vi "lab project final (3).vi"() -> ()   [LabVIEW 2010]
doc: "Use this template to simulate the generation and display of data.\nNote: LabVIEW enables automatic error handling by default for VIs you create from this template."
uses:
  <vilib>/Analysis/4window.llb/windowTd.ctl
  <vilib>/express/express arith-compare/Formula/XNode/ExpressFormulaBlockNode.xnode
  <vilib>/measure/maspectr.llb/FFT Spectrum (Mag-Phase) for 1 Chan.vi
  <vilib>/measure/NI_MAPro.lvlib
  <vilib>/measure/NI_MABase.lvlib
  <vilib>/Analysis/NI_AALPro.lvlib
panel:
  out "Previous":dbl
  out "Result":dbl
  in  "Previous Peak":bool
  in  "Next Peak":bool
  in  "Numeric":dbl
  in  "Span":dbl
  in  "Frequency":dbl
  out "Spectrum Analysis":cluster{"f0":dbl, "df":dbl, "magnitude":dbl[]}(graph)
  in  "Manual Mode":bool
  in  "Number of Cycles":i32(knob) scale=1.0..7.0
  in  "Offset":dbl(knob) scale=0.0..10.0
  in  "signal type":T1(ring)
  in  "Phase":dbl(knob) scale=0.0..10.0
  in  "Frequency":dbl(knob) scale=0.0..10000.0
  in  "Amplitude":dbl(knob) scale=0.0..10.0
  out "Waveform Graph 2":waveform(dbl)(graph)
  in  "window":T2=1 items=["Rectangle"=0, "Hanning"=1, "Hamming"=2, "Blackman-Harris"=3, "Exact Blackman"=4, "Blackman"=5, "Flat Top"=6, "4 Term B-Harris "=7, "7 Term B-Harris"=8, "Low Sidelobe"=9, "Blackman Nuttall"=11, "Triangle"=30, "Bartlett-Hanning"=31, "Bohman"=32, "Parzen"=33, "Welch"=34, "Kaiser"=60, "Dolph-Chebyshev"=61, "Gaussian"=62]
  in  "averaging parameters":T3={"averaging mode"=enum."No averaging", "weighting mode"=enum."Exponential", "number of averages"=10} {"number of averages" min=1}
  out "averaging done":bool
  out "averages completed":dbl
  in  "restart averaging (F)":bool
  in  "view":T4
  in  "stop":bool
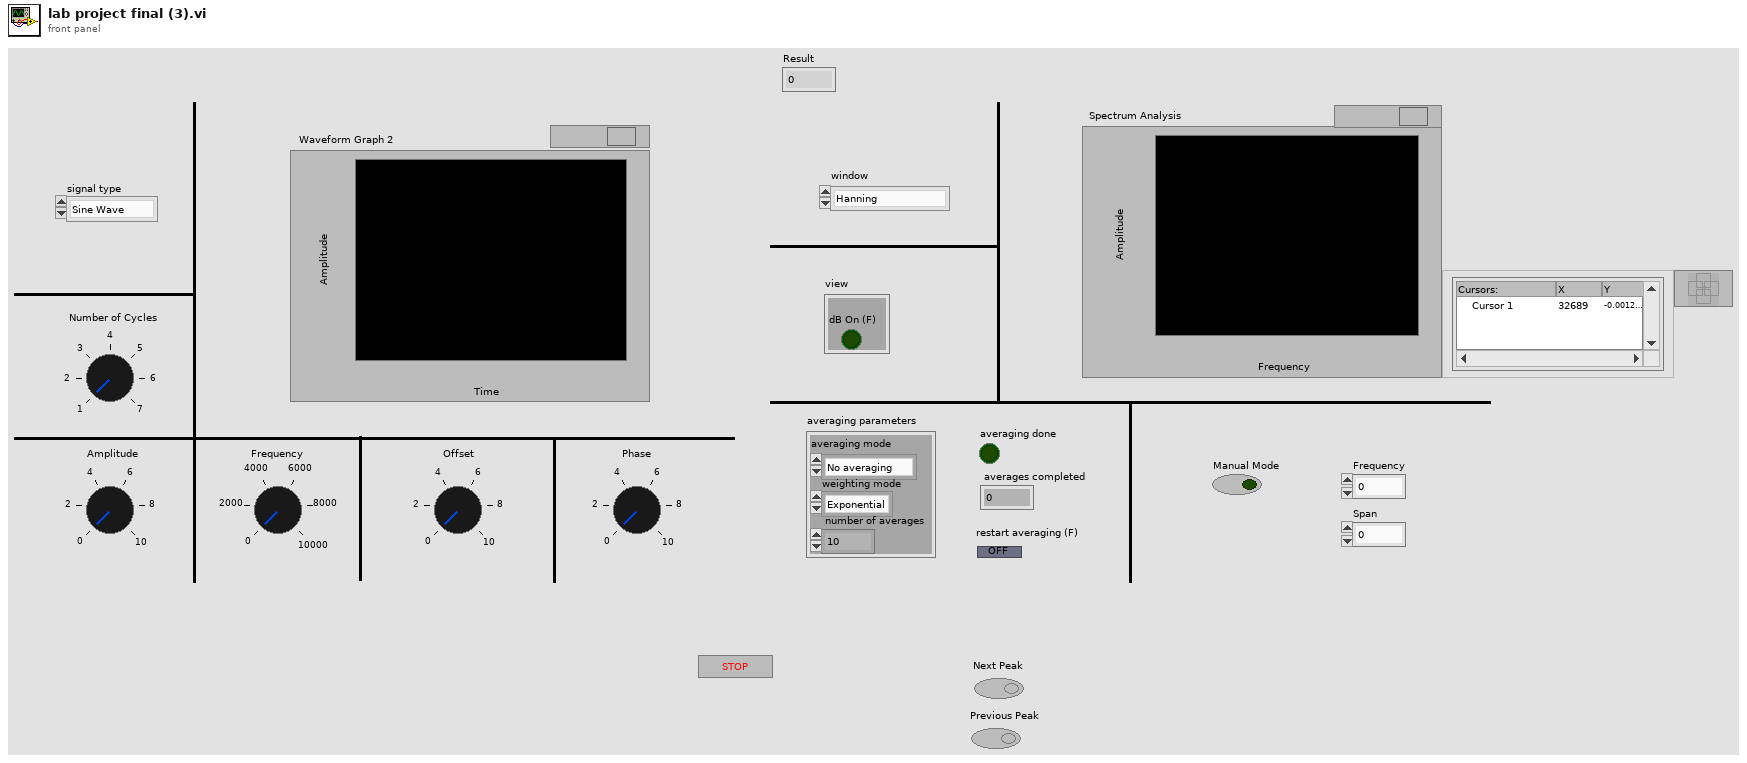
[diagram p1: front panel]
types:
  T1 = enum16{"Sine Wave", "Triangle Wave", "Square Wave", "Sawtooth Wave"}
  T2 = typedef "NI_AALPro.lvlib/windowTd.ctl" = u32
  T3 = cluster{"averaging mode":enum16{"No averaging", "Vector averaging", "RMS averaging", "Peak hold"}, "weighting mode":enum16{"Linear", "Exponential"}, "number of averages":u32}
  T4 = cluster{"dB On (F)":bool, "unwrap phase (F)":bool, "convert to degree (F)":bool}
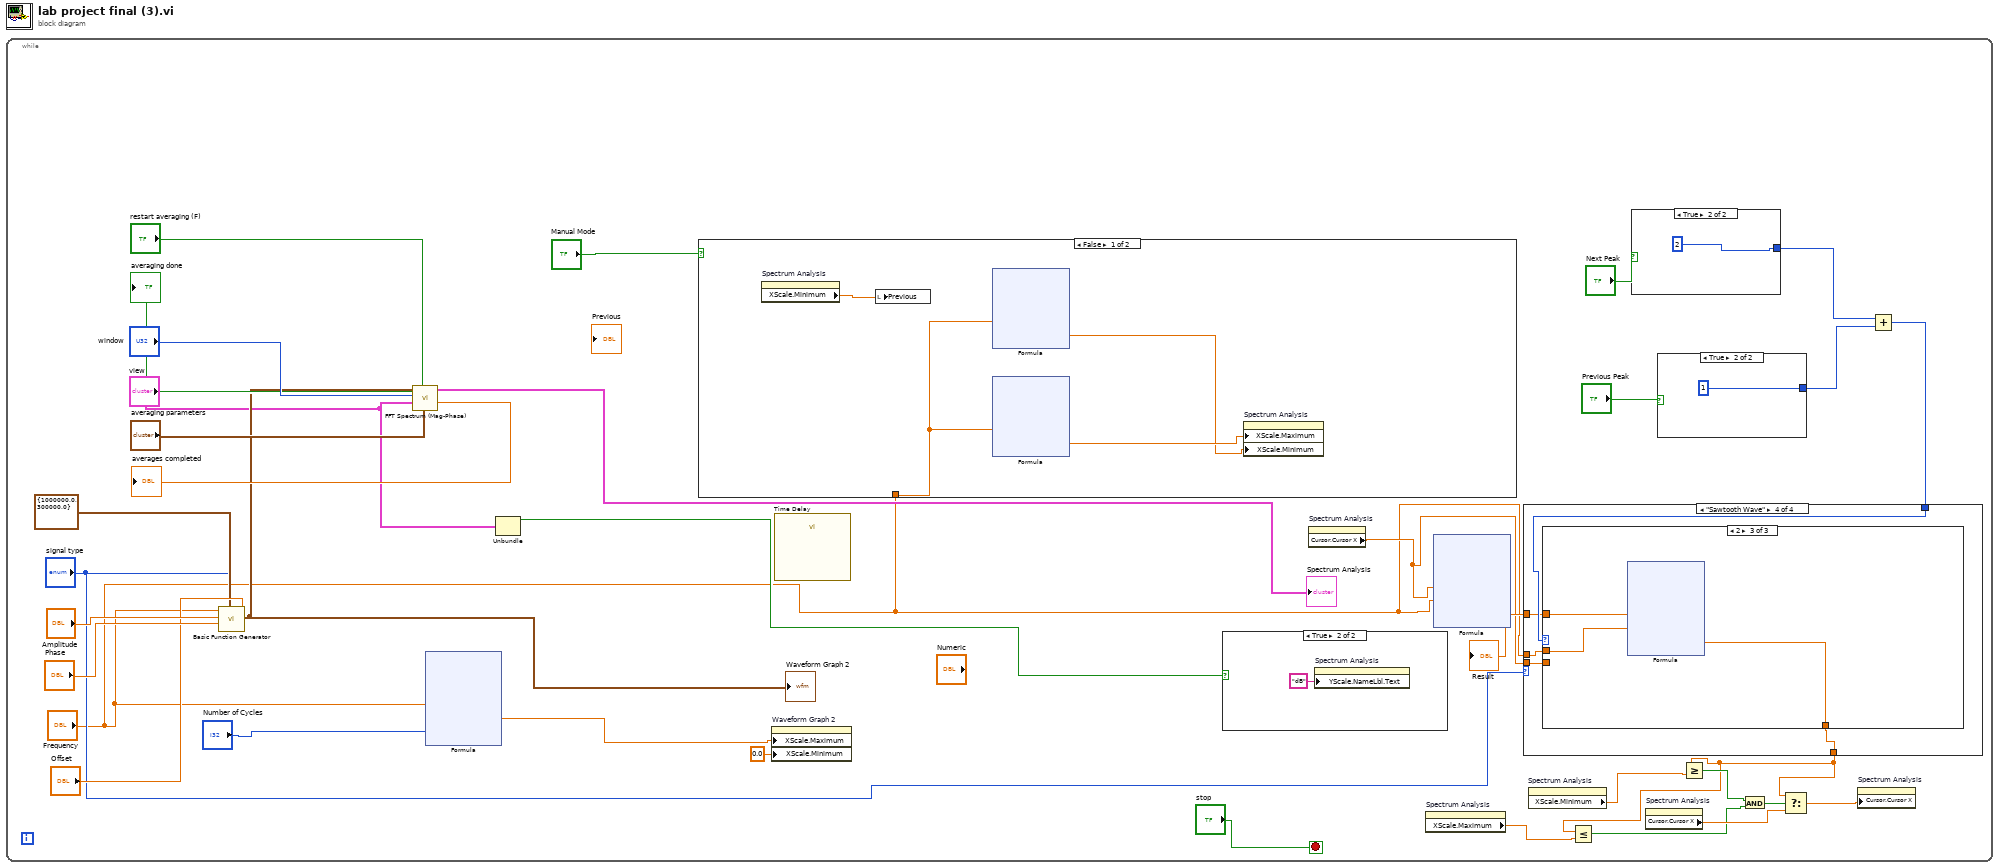
[diagram p0: block diagram]
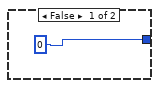
[diagram p2: hidden frame]
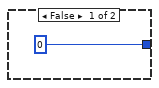
[diagram p3: hidden frame]
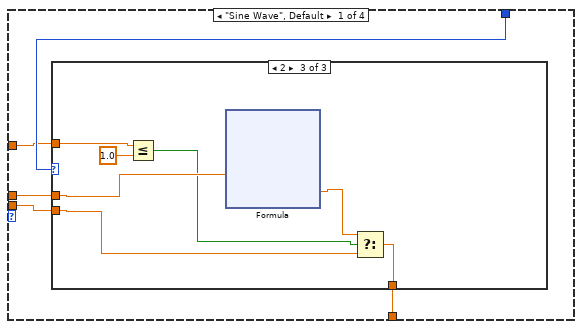
[diagram p4: hidden frame]
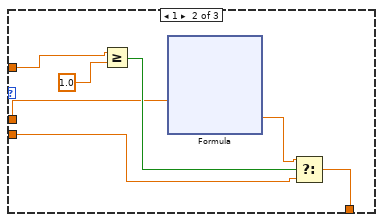
[diagram p6: hidden frame]
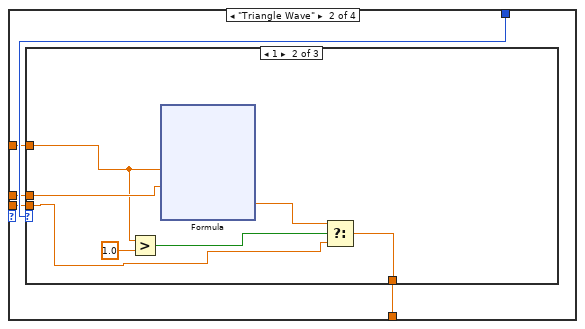
[diagram p7: hidden frame]
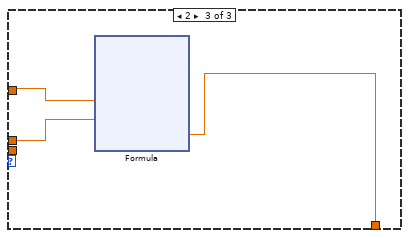
[diagram p9: hidden frame]
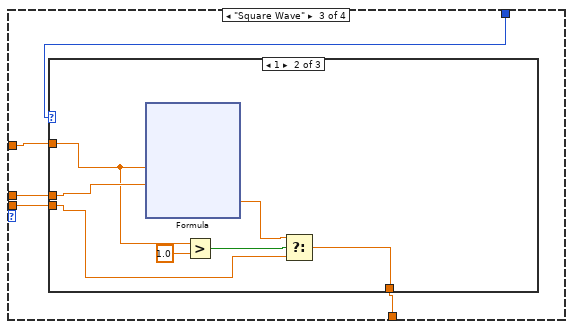
[diagram p10: hidden frame]
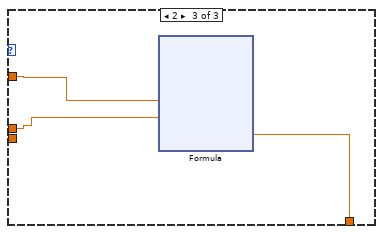
[diagram p12: hidden frame]
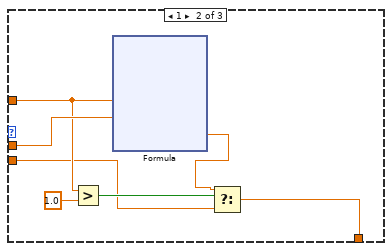
[diagram p14: hidden frame]
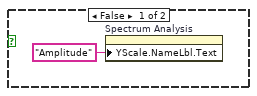
[diagram p15: hidden frame]
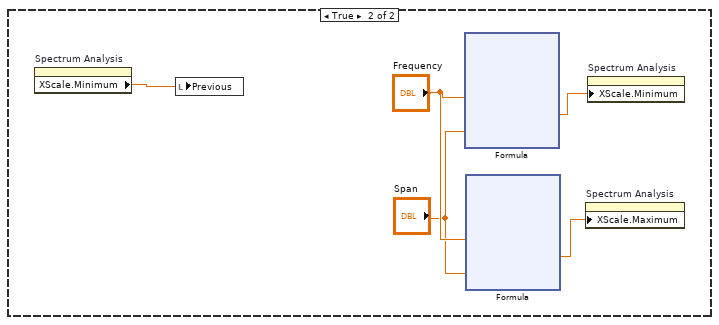
[diagram p16: hidden frame]
diagram:
  n1 = while {
    stop <- "stop" stop-if-true
    n2 = call <vilib>:"Basic Function Generator.vi"("offset"="Offset", "sampling info"=cluster{"Fs":dbl, "#s":dbl} {"Fs"=1000000.0, "#s"=300000.0}, "signal type"="signal type", "phase"="Phase", "amplitude"="Amplitude", "frequency"="Frequency") -> ("signal out"=w24:waveform(dbl))  [unwired: 3 in, 2 out]
    "Waveform Graph 2" <- w24
    n3 = call-poly <vilib>:"FFT Spectrum (Mag-Phase).vi"("averaging parameters"="averaging parameters", "restart averaging (F)"="restart averaging (F)", "view"="view", "window"="window", "time signal"=w24) -> ("averages completed"=→"averages completed":dbl, "magnitude"=→"Spectrum Analysis":cluster{"f0":dbl, "df":dbl, "magnitude":dbl[]}, "averaging done"=→"averaging done":bool)  [unwired: 2 in, 2 out]
    n4 = xnode "Formula"("frequency"="Frequency", "n"="Number of Cycles") -> ("Result"=w20:dbl)  [unwired: 1 in, 1 out]
    n5 = Unbundle("view") -> ("dB On (F)"=w22:bool)  [unwired: 2 out]
    n6 = case shown="False" "Manual Mode" {
      tunnel: "Frequency" -> [w209 _]
      frame False {
        n7 = property on="Spectrum Analysis" class="WFGraph (strict)"() -> ("XScale.Minimum"=w206:dbl)  [unwired: 2 in, 2 out]
        n8 = local write "Previous"(w206) -> ()
        n9 = xnode "Formula"("frequency"=w209) -> ("Result"=w207:dbl)  [unwired: 1 in, 1 out]
        n10 = xnode "Formula"("frequency"=w209) -> ("Result"=w208:dbl)  [unwired: 1 in, 1 out]
        n11 = property on="Spectrum Analysis" class="WFGraph (strict)"("XScale.Maximum"=w208, "XScale.Minimum"=w207) -> ()  [unwired: 2 in, 2 out]
      }
      frame True {
        n12 = property on="Spectrum Analysis" class="WFGraph (strict)"() -> ("XScale.Minimum"=w226:dbl)  [unwired: 2 in, 2 out]
        n13 = local write "Previous"(w226) -> ()
        n14 = xnode "Formula"("frequency"="Frequency", "span"="Span") -> ("Result"=w230:dbl)  [unwired: 1 in, 1 out]
        n15 = xnode "Formula"("frequency"="Frequency", "span"="Span") -> ("Result"=w229:dbl)  [unwired: 1 in, 1 out]
        n16 = property on="Spectrum Analysis" class="WFGraph (strict)"("XScale.Maximum"=w229) -> ()  [unwired: 2 in, 2 out]
        n17 = property on="Spectrum Analysis" class="WFGraph (strict)"("XScale.Minimum"=w230) -> ()  [unwired: 2 in, 2 out]
      }
    }
    n18 = property on="Waveform Graph 2" class="WFGraph (strict)"("XScale.Maximum"=w20, "XScale.Minimum"=0.0 ("X Scale.Range:Minimum")) -> ()  [unwired: 2 in, 2 out]
    n19 = call "Time Delay"() -> ()  [unwired: 11 in, 1 out]
    n20 = case shown="True" w22 {
      frame False {
        n21 = property on="Spectrum Analysis" class="WFGraph (strict)"("YScale.NameLbl.Text"="Amplitude" ("Y Scale.Name Label.Text")) -> ()  [unwired: 2 in, 2 out]
      }
      frame True {
        n22 = property on="Spectrum Analysis" class="WFGraph (strict)"("YScale.NameLbl.Text"="dB" ("Y Scale.Name Label.Text")) -> ()  [unwired: 2 in, 2 out]
      }
    }
    n23 = property on="Spectrum Analysis" class="WFGraph (strict)"() -> ("Cursor.Cursor X"=w10:dbl)  [unwired: 2 in, 2 out]
    n24 = property on="Spectrum Analysis" class="WFGraph (strict)"() -> ("XScale.Maximum"=w3:dbl)  [unwired: 2 in, 2 out]
    n25 = xnode "Formula"("POS"=w10, "FREQ"="Frequency") -> ("Result"=w11:dbl)  [unwired: 1 in, 1 out]
    "Result" <- w11
    n26 = property on="Spectrum Analysis" class="WFGraph (strict)"() -> ("XScale.Minimum"=w4:dbl)  [unwired: 2 in, 2 out]
    n27 = case shown="True" "Next Peak" {
      tunnel: [0 2] -> w14
      frame False {
      }
      frame True {
      }
    }
    n28 = property on="Spectrum Analysis" class="WFGraph (strict)"() -> ("Cursor.Cursor X"=w6:dbl)  [unwired: 2 in, 2 out]
    n29 = case shown="True" "Previous Peak" {
      tunnel: [0 1] -> w13
      frame False {
      }
      frame True {
      }
    }
    n30 = Add(x=w14, y=w13) -> (x+y=w12:i32)
    n31 = case shown="\"Sawtooth Wave\"" "signal type" {
      tunnel: w12 -> [w54 w90 w126 w162]
      tunnel: w11 -> [w53 w89 w123 w159]
      tunnel: [w51 w88 w124 w160] -> w2
      tunnel: w10 -> [w52 w86 w125 w161]
      tunnel: "Frequency" -> [w50 w87 w122 w158]
      frame "Sine Wave", Default {
        n32 = case shown="2" w54 {
          tunnel: w53 -> [_ w62 w77]
          tunnel: w52 -> [w55 w56 w71]
          tunnel: [w55 w60 w75] -> w51
          tunnel: w50 -> [_ w57 w74]
          frame 0, Default {
          }
          frame 1 {
            n33 = Greater Or Equal?(x=w62, y=1.0) -> (x >= y?=w59:bool)
            n34 = xnode "Formula"("Freq"=w57) -> ("Result"=w58:dbl)  [unwired: 1 in, 1 out]
            n35 = Select(t=w58, s=w59, f=w56) -> (s? t:f=w60:dbl)
          }
          frame 2 {
            n36 = Less Or Equal?(x=w77, y=1.0) -> (x <= y?=w73:bool)
            n37 = xnode "Formula"("Freq"=w74) -> ("Result"=w72:dbl)  [unwired: 1 in, 1 out]
            n38 = Select(t=w72, s=w73, f=w71) -> (s? t:f=w75:dbl)
          }
        }
      }
      frame "Triangle Wave" {
        n39 = case shown="1" w90 {
          tunnel: w89 -> [_ w95 w111]
          tunnel: [w91 w92 w110] -> w88
          tunnel: w87 -> [_ w98 w109]
          tunnel: w86 -> [w91 w93 _]
          frame 0, Default {
          }
          frame 1 {
            n40 = Greater?(x=w95, y=1.0) -> (0:w94:bool)
            n41 = xnode "Formula"("Input"=w95, "Freq"=w98) -> ("Result"=w97:dbl)  [unwired: 1 in, 1 out]
            n42 = Select(t=w97, s=w94, f=w93) -> (s? t:f=w92:dbl)
          }
          frame 2 {
            n43 = xnode "Formula"("Input"=w111, "Freq"=w109) -> ("Result"=w110:dbl)  [unwired: 1 in, 1 out]
          }
        }
      }
      frame "Square Wave" {
        n44 = case shown="1" w126 {
          tunnel: [w127 w129 w147] -> w124
          tunnel: w125 -> [w127 w128 _]
          tunnel: w123 -> [_ w130 w146]
          tunnel: w122 -> [_ w134 w145]
          frame 0, Default {
          }
          frame 1 {
            n45 = xnode "Formula"("Input"=w130, "Freq"=w134) -> ("Result"=w131:dbl)  [unwired: 1 in, 1 out]
            n46 = Greater?(x=w130, y=1.0) -> (0:w132:bool)
            n47 = Select(t=w131, s=w132, f=w128) -> (s? t:f=w129:dbl)
          }
          frame 2 {
            n48 = xnode "Formula"("Input"=w146, "Freq"=w145) -> ("Result"=w147:dbl)  [unwired: 1 in, 1 out]
          }
        }
      }
      frame "Sawtooth Wave" {
        n49 = case shown="2" w162 {
          tunnel: [w163 w166 w181] -> w160
          tunnel: w161 -> [w163 w164 _]
          tunnel: w159 -> [_ w169 w183]
          tunnel: w158 -> [_ w170 w182]
          frame 0, Default {
          }
          frame 1 {
            n50 = Greater?(x=w169, y=1.0) -> (0:w167:bool)
            n51 = xnode "Formula"("Input"=w169, "Freq"=w170) -> ("Result"=w165:dbl)  [unwired: 1 in, 1 out]
            n52 = Select(t=w165, s=w167, f=w164) -> (s? t:f=w166:dbl)
          }
          frame 2 {
            n53 = xnode "Formula"("Input"=w183, "Freq"=w182) -> ("Result"=w181:dbl)  [unwired: 1 in, 1 out]
          }
        }
      }
    }
    n54 = Less Or Equal?(x=w2, y=w3) -> (x <= y?=w1:bool)
    n55 = Greater Or Equal?(x=w2, y=w4) -> (x >= y?=w5:bool)
    n56 = And(x=w5, y=w1) -> (x .and. y?=w8:bool)
    n57 = Select(t=w2, s=w8, f=w6) -> (s? t:f=w7:dbl)
    n58 = property on="Spectrum Analysis" class="WFGraph (strict)"("Cursor.Cursor X"=w7) -> ()  [unwired: 2 in, 2 out]
  }
